vi "仁科测控通讯.vi"() -> ()   [LabVIEW 2016, in "环境动力监测库.lvlib" / "空调库.lvlib"]
uses:
  <vilib>/Plasmionique/MB Master/MB_Master/MB_Master.lvclass
  <vilib>/Plasmionique/MB Master/MB Master.lvlib
panel:
  out "运行状态":T1
  out "告警状态":T2
  out "传感器状态输出":T3
  out "温湿度解析":cluster{"湿度":dbl, "温度":dbl}
  out "系统参数":u16[](array[numeric])
  out "告警状态":u16[](array[numeric])
  out "传感器状态":u16[](array[numeric])
  out "温湿度解析":u16[](array[numeric])
  in  "读取数据":bool
  in  "释放串口":bool
  in  "打开串口":bool
  out "通讯状态":bool
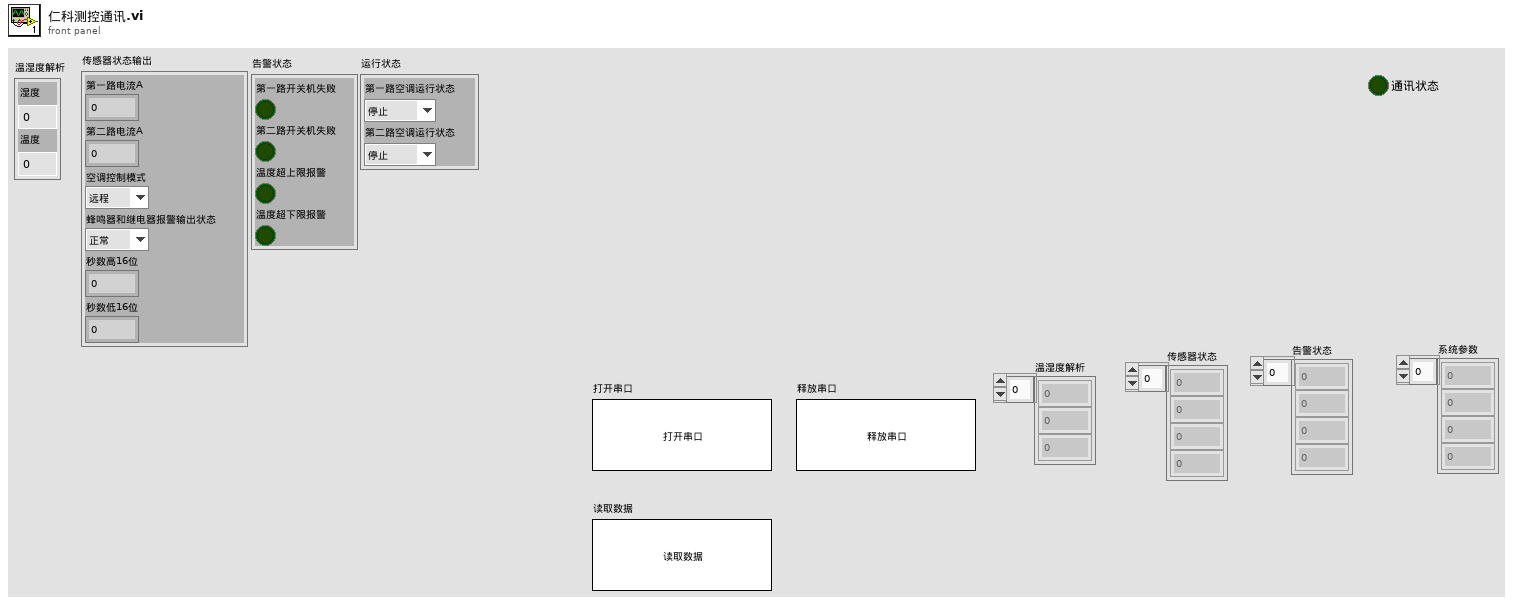
[diagram p1: front panel]
types:
  T1 = cluster{"第一路空调运行状态":enum16{"停止", "制冷", "制热", "未知"}, "第二路空调运行状态":enum16{"停止", "制冷", "制热", "未知"}}
  T2 = cluster{"第一路开关机失败":bool, "第二路开关机失败":bool, "温度超上限报警":bool, "温度超下限报警":bool}
  T3 = cluster{"第一路电流A":u16, "第二路电流A":u16, "空调控制模式":enum16{"远程", "自动"}, "蜂鸣器和继电器报警输出状态":enum16{"正常", "报警"}, "秒数高16位":u16, "秒数低16位":u16}
  T4 = cluster{"型号选择":enum16{"黑盾", "英维克", "仁科测控RS-KTC-N01"}, "MB session in":refnum<class "MB_Master.lvclass">, "英维克空调寄存器":u16[], "通讯状态":bool, "PORT":string, "IP":string, "Slave ID ":u8, "Serial Config":cluster{"baud rate (bps)":u32, "stop bits":u16, "parity":u16, "flow control":u16, "timeout":u32, "retries":i32}, "VISA Resource":refnum<visa-resource-name>, "MB通信方式选择":enum16{"串口", "TCP"}}
  T5 = enum16{"open", "read", "write single", "write", "close"}
  T6 = cluster{"温湿度解析":cluster{"湿度":dbl, "温度":dbl}, "传感器状态输出":cluster{"第一路电流A":u16, "第二路电流A":u16, "空调控制模式":enum16{"远程", "自动"}, "蜂鸣器和继电器报警输出状态":enum16{"正常", "报警"}, "秒数高16位":u16, "秒数低16位":u16}, "告警状态":cluster{"第一路开关机失败":bool, "第二路开关机失败":bool, "温度超上限报警":bool, "温度超下限报警":bool}, "运行状态":cluster{"第一路空调运行状态":enum16{"停止", "制冷", "制热", "未知"}, "第二路空调运行状态":enum16{"停止", "制冷", "制热", "未知"}}}
  T7 = cluster{"第一路电流":u16, "第二路电流":u16, "空调控制模式":enum16{"远程", "自动"}, "蜂鸣器和继电器报警输出状态":enum16{"正常", "报警"}, "秒数高16位":u16, "秒数低16位":u16}
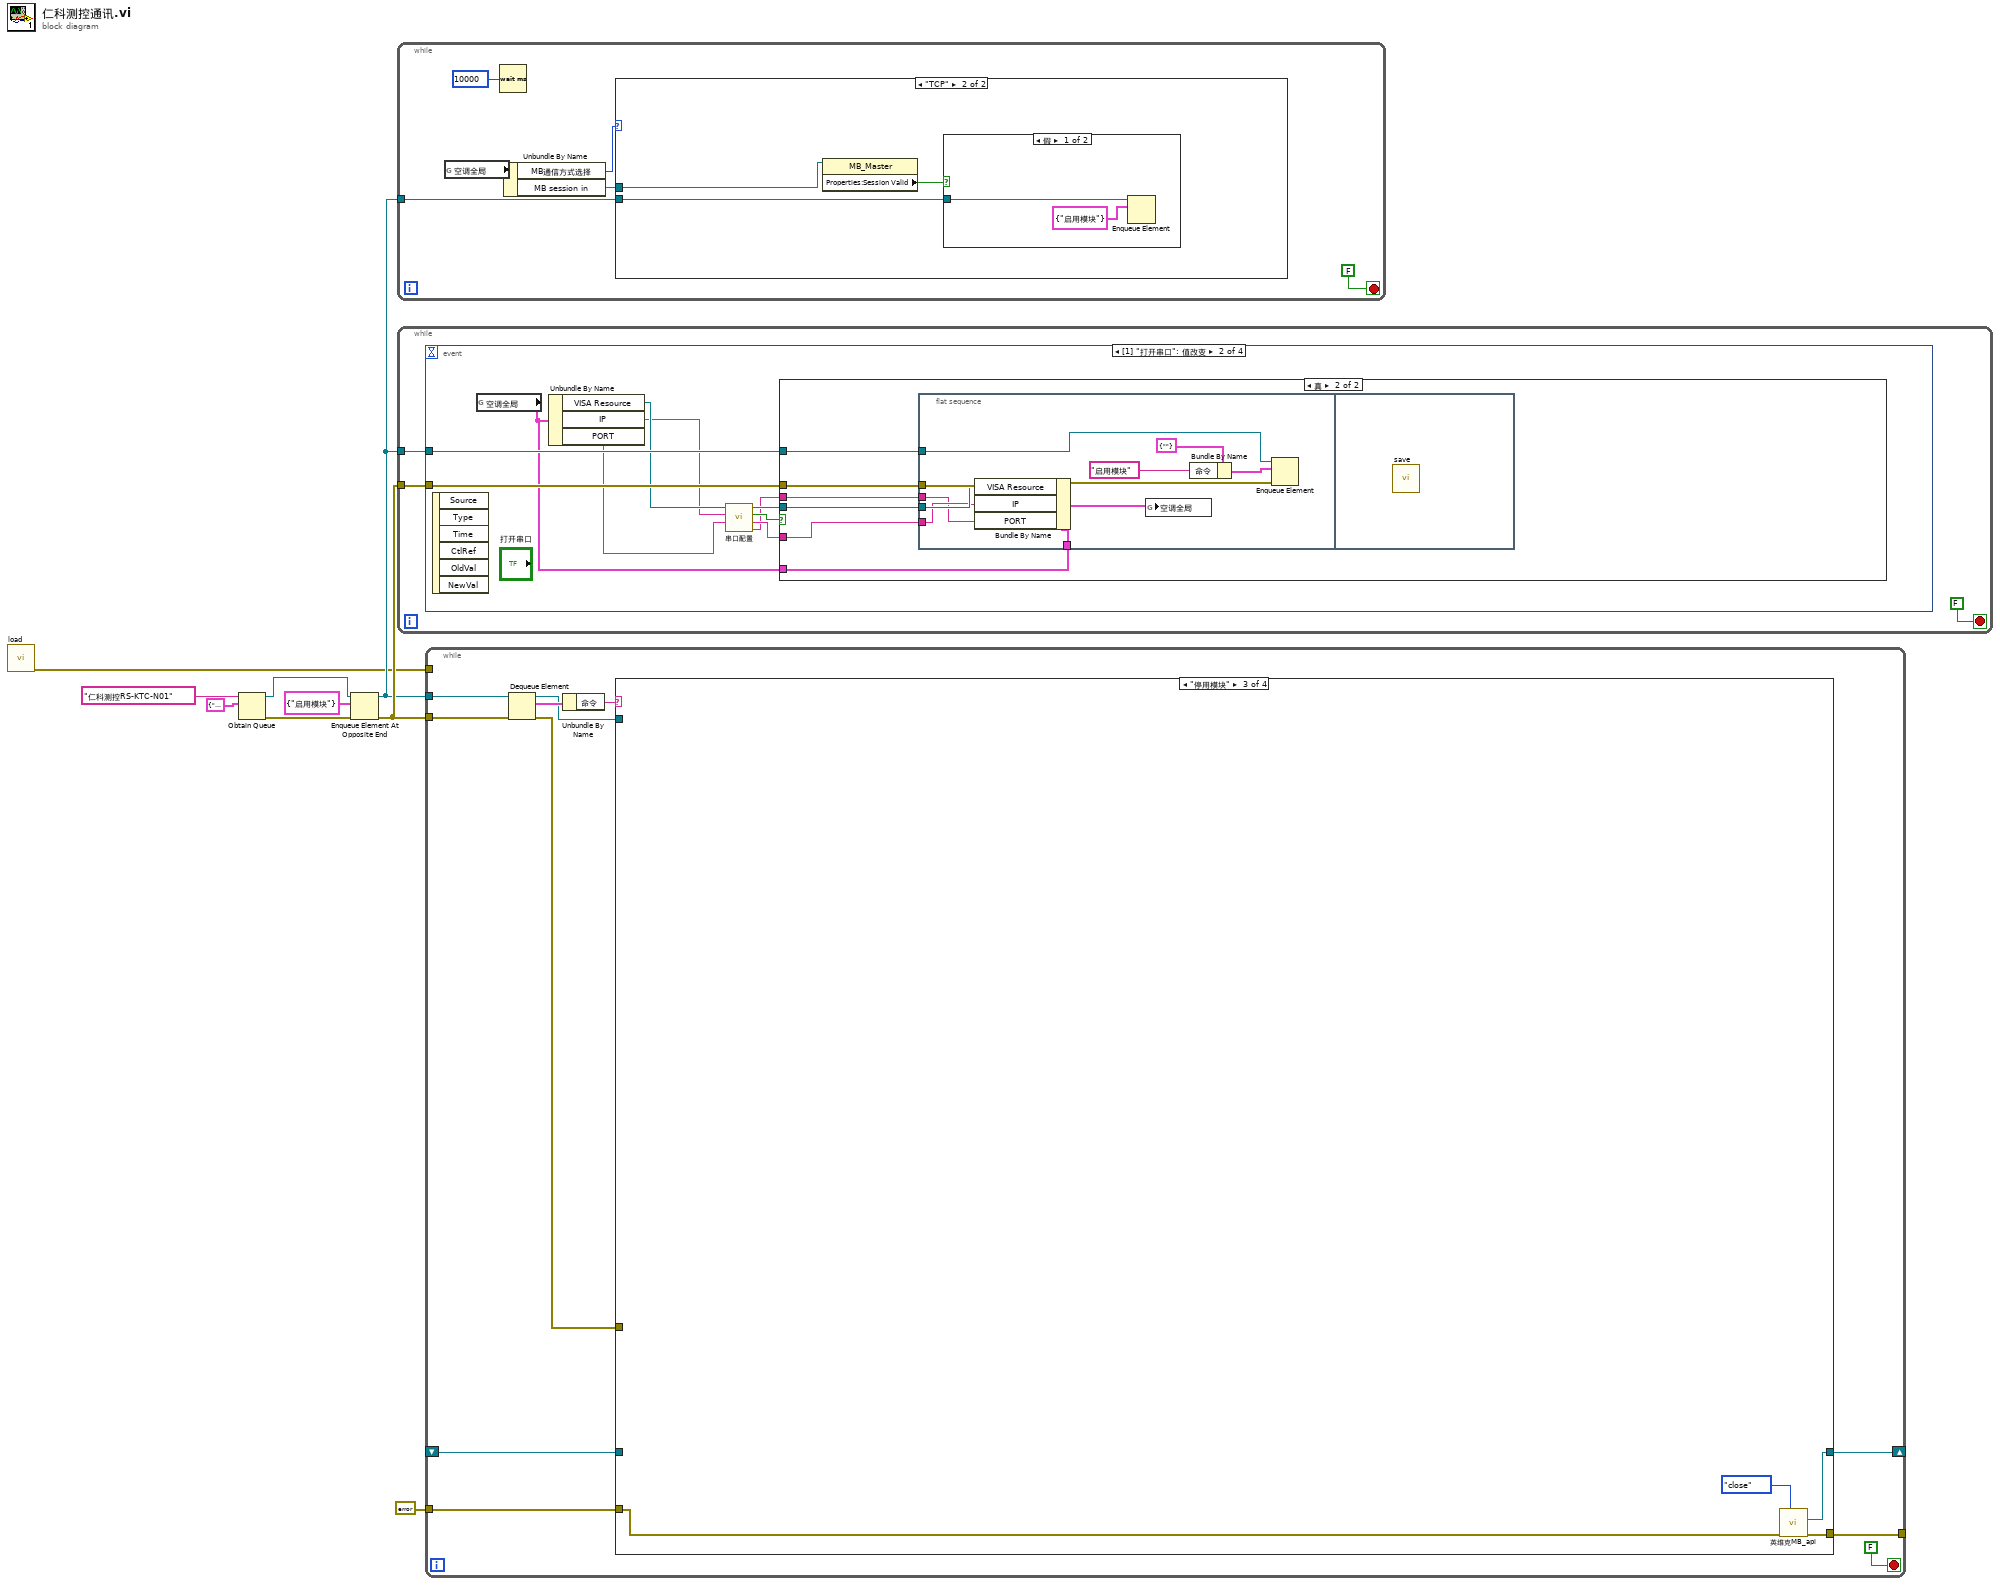
[diagram p0: block diagram]
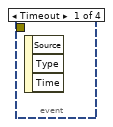
[diagram p4: hidden frame]
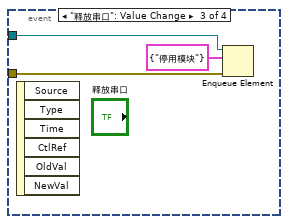
[diagram p6: hidden frame]
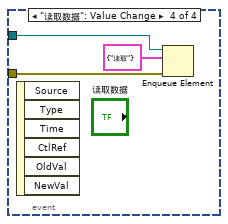
[diagram p7: hidden frame]
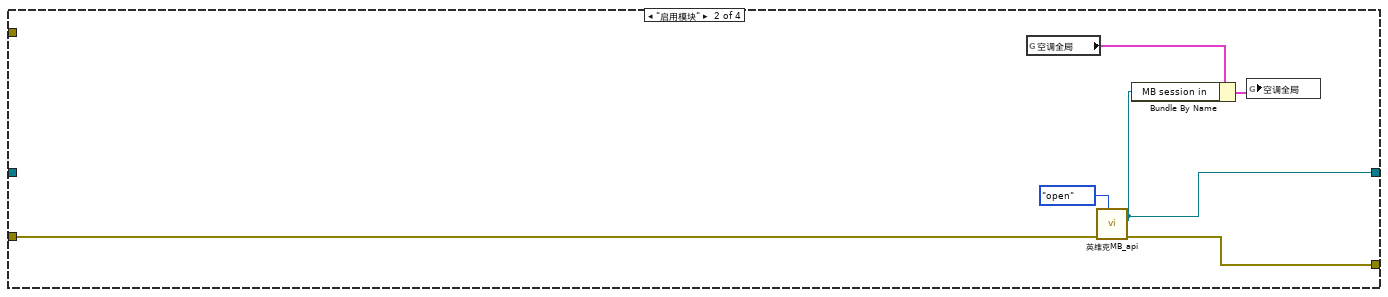
[diagram p9: hidden frame]
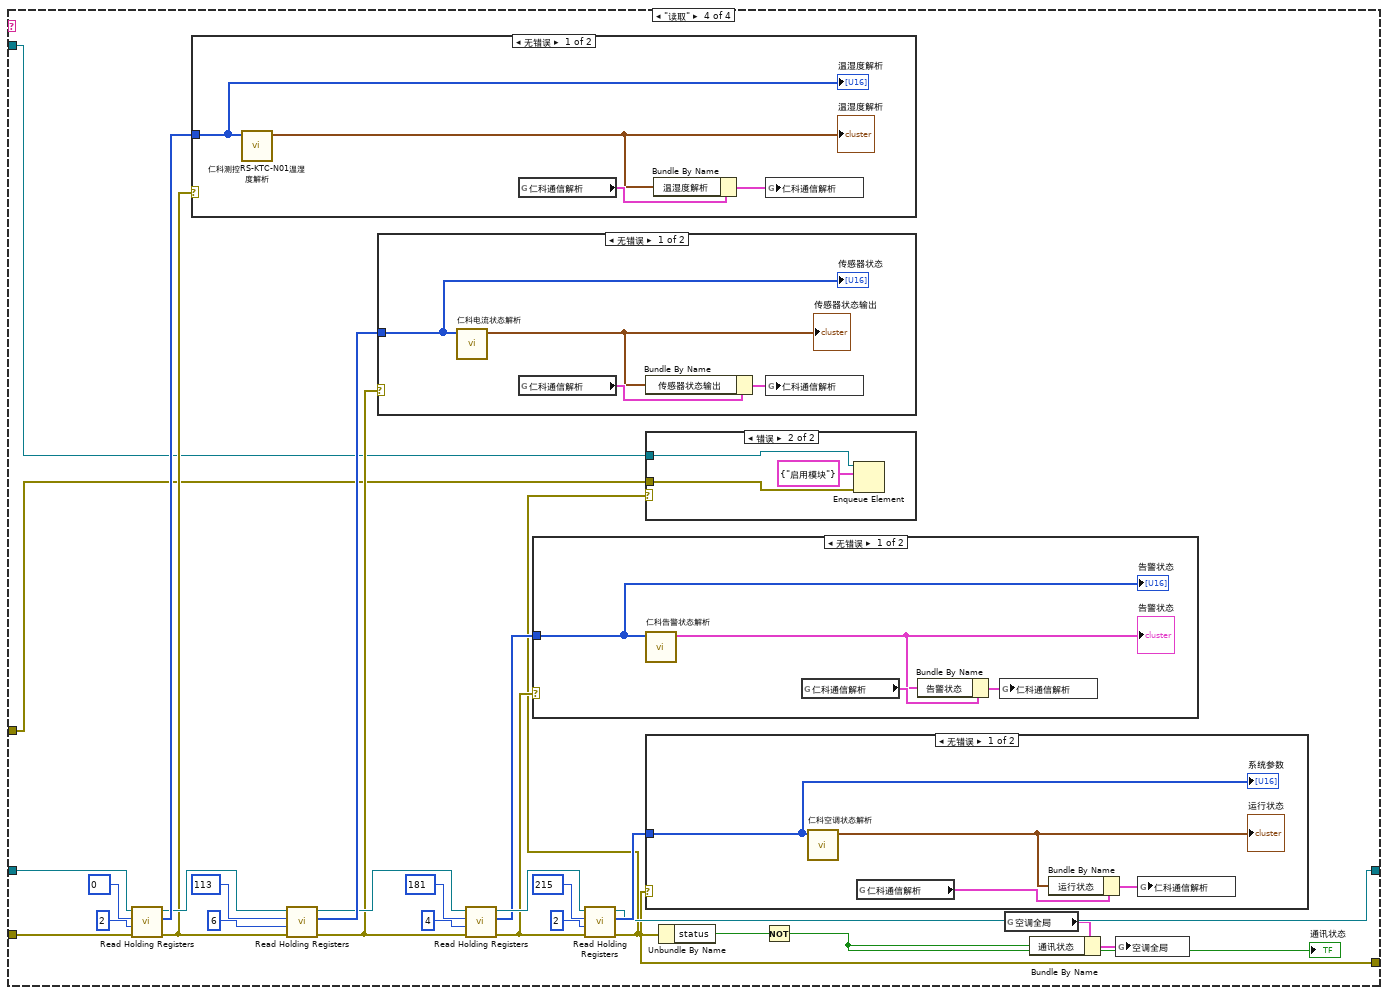
[diagram p10: hidden frame]
diagram:
  n1 = call "load.vi"() -> ("error out"=w1:errorcluster)  [unwired: 11 in]
  n2 = Obtain Queue(name (unnamed)="仁科测控RS-KTC-N01" ("名称（未命名）"), element data type=cluster{"命令":string} {"命令"="启用模块"} ("元素")) -> (queue out=w6:refnum<queue>, error out=w5:errorcluster)  [unwired: 3 in, 1 out]
  n3 = Enqueue Element At Opposite End(queue=w6, element=cluster{"命令":string} {"命令"="启用模块"} ("元素"), error in (no error)=w5) -> (queue out=w2:refnum<queue>, error out=w3:errorcluster)  [unwired: 1 in, 1 out]
  n4 = while {
    tunnel: w2 -> [w15]
    stop <- FALSE stop-if-true
    n5 = global read "断电保存全局变量.vi" "空调全局"() -> (w12:T4)
    n6 = Wait (ms)(milliseconds to wait=u32 10000 ("等待时间（毫秒）")) -> ()  [unwired: 1 out]
    n7 = Unbundle By Name(w12) -> ("MB通信方式选择"=w11:enum16{"串口", "TCP"}, "MB session in"=w10:refnum<class "MB_Master.lvclass">)
    n8 = case shown="\"TCP\"" w11 {
      tunnel: w15 -> [_ w17]
      tunnel: w10 -> [_ w16]
      frame "串口", Default {
      }
      frame "TCP" {
        n9 = property class="MB_Master"(reference=w16) -> ("Properties:Session Valid"=w18:bool)  [unwired: 1 in, 2 out]
        n10 = case shown="假" w18 {
          tunnel: w17 -> [w20 _]
          frame False {
            n11 = Enqueue Element(queue=w20, element=cluster{"命令":string} {"命令"="启用模块"} ("元素")) -> ()  [unwired: 2 in, 3 out]
          }
          frame True {
          }
        }
      }
    }
  }
  n12 = while {
    tunnel: w2 -> [w22]
    tunnel: w3 -> [w21]
    stop <- FALSE stop-if-true
    n13 = event shown="[1] \"打开串口\": 值改变" {
      selector: _ -> [_ _ _ _]
      dyn-events: _ -> [_ _ _ _]
      timeout: _ -> [_ _ _ _]
      tunnel: w22 -> [_ w33 w52 w54]
      tunnel: w21 -> [_ w32 w51 w53]
      event Timeout {
        n14 = event-data() -> ()  [unwired: 1 in, 3 out]
      }
      event "打开串口": Value Change {
        n15 = event-data() -> ()  [unwired: 1 in, 6 out]
        n16 = global read "断电保存全局变量.vi" "空调全局"() -> (w24:T4)
        n17 = Unbundle By Name(w24) -> ("VISA Resource"=w27:refnum<visa-resource-name>, "IP"=w26:string, "PORT"=w25:string)
        n18 = call "串口配置.vi"("PORT"=w25, "IP"=w26, "请选择串口:"=w27) -> ("PORT 2"=w28:string, "IP 2"=w29:string, "确认 2"=w30:bool, "VISA资源名称 2"=w31:refnum<visa-resource-name>)  [unwired: 5 in]
        n19 = case shown="真" w30 {
          tunnel: w31 -> [_ w37]
          tunnel: w33 -> [_ w39]
          tunnel: w32 -> [_ w38]
          tunnel: w29 -> [_ w36]
          tunnel: w28 -> [_ w35]
          tunnel: w24 -> [_ w34]
          frame False {
          }
          frame True {
            n20 = flat-sequence {
              tunnel: w39 -> [w46]
              tunnel: w38 -> [w45]
              tunnel: w37 -> [w42]
              tunnel: w36 -> [w41]
              tunnel: w35 -> [w40]
              tunnel: w34 -> [w44]
              frame #0 {
                n21 = Bundle By Name(cluster=w44, "VISA Resource"=w42, "IP"=w41, "PORT"=w40) -> (w43:T4)
                n22 = global write "断电保存全局变量.vi" "空调全局"(w43) -> ()
                n23 = Bundle By Name(cluster=cluster{"命令":string} {"命令"=""} ("元素"), "命令"="启用模块" ("名称（未命名）")) -> (w47:cluster{"命令":string})
                n24 = Enqueue Element(queue=w46, element=w47, error in (no error)=w45) -> ()  [unwired: 1 in, 3 out]
              }
              frame #1 {
                n25 = call "save.vi"() -> ()  [unwired: 11 in, 1 out]
              }
            }
          }
        }
      }
      event "释放串口": Value Change {
        n26 = event-data() -> ()  [unwired: 1 in, 6 out]
        n27 = Enqueue Element(queue=w52, element=cluster{"命令":string} {"命令"="停用模块"} ("元素"), error in (no error)=w51) -> ()  [unwired: 1 in, 3 out]
      }
      event "读取数据": Value Change {
        n28 = event-data() -> ()  [unwired: 1 in, 6 out]
        n29 = Enqueue Element(queue=w54, element=cluster{"命令":string} {"命令"="读取"} ("元素"), error in (no error)=w53) -> ()  [unwired: 1 in, 3 out]
      }
    }
  }
  n30 = while {
    tunnel: w2 -> [w58]
    tunnel: w3 -> [w65]
    tunnel: [w59] -> _
    shift-right: [w62] -> _
    shift-left: _ -> [w61]
    tunnel: errorcluster {"status"=FALSE, "code"=0, "source"=""} ("error out") -> [w60]
    tunnel: w1 -> [_]
    stop <- FALSE stop-if-true
    n31 = Dequeue Element(queue=w58, error in (no error)=w65) -> (queue out=w57:refnum<queue>, element=w64:cluster{"命令":string}, error out=w56:errorcluster)  [unwired: 1 in, 1 out]
    n32 = Unbundle By Name(w64) -> ("命令"=w63:string)
    n33 = case shown="\"停用模块\"" w63 {
      tunnel: [w68 w70 w76 w83] -> w62
      tunnel: [w67 w74 w77 w82] -> w59
      tunnel: w61 -> [w68 _ _ w106]
      tunnel: w60 -> [w67 w73 w78 w105]
      tunnel: w57 -> [_ _ _ w85]
      tunnel: w56 -> [_ _ _ w84]
      frame Default {
      }
      frame "启用模块" {
        n34 = global read "断电保存全局变量.vi" "空调全局"() -> (w71:T4)
        n35 = call "英维克MB_api.vi"("STEP"=T5."open", "Error in"=w73) -> ("error out"=w74:errorcluster, "MB session out"=w70:refnum<class "MB_Master.lvclass">)  [unwired: 7 in, 1 out]
        n36 = Bundle By Name(cluster=w71, "MB session in"=w70) -> (w69:T4)
        n37 = global write "断电保存全局变量.vi" "空调全局"(w69) -> ()
      }
      frame "停用模块" {
        n38 = call "英维克MB_api.vi"("STEP"=T5."close", "Error in"=w78) -> ("error out"=w77:errorcluster, "MB session out"=w76:refnum<class "MB_Master.lvclass">)  [unwired: 7 in, 1 out]
      }
      frame "读取" {
        n39 = call <vilib>:"Read Holding Registers.vi"("error in (no error)"=w105, "quantity"=u16 2 ("number of holding registers"), "starting address"=u16 0, "MB session in"=w106) -> ("error out"=w102:errorcluster, "Registers"=w104:u16[], "MB session out"=w103:refnum<class "MB_Master.lvclass">)  [unwired: 5 in]
        n40 = case shown="无错误" w102 {
          tunnel: w104 -> [w125 _]
          frame No Error {
            n41 = call "仁科测控RS-KTC-N01温湿度解析.vi"("运行状态输入"=w125) -> ("温湿度解析"=w122:cluster{"湿度":dbl, "温度":dbl})  [unwired: 10 in]
            "温湿度解析" <- w122
            n42 = global read "内部交互全局变量.vi" "仁科通信解析"() -> (w124:T6)
            n43 = Bundle By Name(cluster=w124, "温湿度解析"=w122) -> (w123:T6)
            n44 = global write "内部交互全局变量.vi" "仁科通信解析"(w123) -> ()
            "温湿度解析" <- w125
          }
          frame Error {
          }
        }
        n45 = call <vilib>:"Read Holding Registers.vi"("error in (no error)"=w102, "quantity"=u16 6 ("number of holding registers"), "starting address"=u16 113, "MB session in"=w103) -> ("error out"=w94:errorcluster, "Registers"=w101:u16[], "MB session out"=w95:refnum<class "MB_Master.lvclass">)  [unwired: 5 in]
        n46 = case shown="无错误" w94 {
          tunnel: w101 -> [w121 _]
          frame No Error {
            n47 = call "仁科电流状态解析.vi"("传感器状态输入"=w121) -> ("传感器状态输出"=w118:T7)  [unwired: 10 in]
            "传感器状态输出" <- w118
            n48 = global read "内部交互全局变量.vi" "仁科通信解析"() -> (w120:T6)
            n49 = Bundle By Name(cluster=w120, "传感器状态输出"=w118) -> (w119:T6)
            n50 = global write "内部交互全局变量.vi" "仁科通信解析"(w119) -> ()
            "传感器状态" <- w121
          }
          frame Error {
          }
        }
        n51 = call <vilib>:"Read Holding Registers.vi"("error in (no error)"=w94, "quantity"=u16 4 ("number of holding registers"), "starting address"=u16 181, "MB session in"=w95) -> ("error out"=w88:errorcluster, "Registers"=w87:u16[], "MB session out"=w89:refnum<class "MB_Master.lvclass">)  [unwired: 5 in]
        n52 = case shown="无错误" w88 {
          tunnel: w87 -> [w117 _]
          frame No Error {
            n53 = call "仁科告警状态解析.vi"("告警状态输入"=w117) -> ("告警状态"=w114:T2)  [unwired: 10 in]
            "告警状态" <- w114
            n54 = global read "内部交互全局变量.vi" "仁科通信解析"() -> (w116:T6)
            n55 = Bundle By Name(cluster=w116, "告警状态"=w114) -> (w115:T6)
            n56 = global write "内部交互全局变量.vi" "仁科通信解析"(w115) -> ()
            "告警状态" <- w117
          }
          frame Error {
          }
        }
        n57 = call <vilib>:"Read Holding Registers.vi"("error in (no error)"=w88, "quantity"=u16 2 ("number of holding registers"), "starting address"=u16 215, "MB session in"=w89) -> ("error out"=w82:errorcluster, "Registers"=w86:u16[], "MB session out"=w83:refnum<class "MB_Master.lvclass">)  [unwired: 5 in]
        n58 = case shown="错误" w82 {
          tunnel: w85 -> [_ w109]
          tunnel: w84 -> [_ w107]
          frame No Error {
          }
          frame Error {
            n59 = Enqueue Element(queue=w109, element=cluster{"命令":string} {"命令"="启用模块"} ("元素"), error in (no error)=w107) -> ()  [unwired: 1 in, 3 out]
          }
        }
        n60 = case shown="无错误" w82 {
          tunnel: w86 -> [w113 _]
          frame No Error {
            n61 = call "仁科空调状态解析.vi"("系统参数输入"=w113) -> ("运行状态"=w110:T1)  [unwired: 10 in]
            "运行状态" <- w110
            n62 = global read "内部交互全局变量.vi" "仁科通信解析"() -> (w112:T6)
            n63 = Bundle By Name(cluster=w112, "运行状态"=w110) -> (w111:T6)
            n64 = global write "内部交互全局变量.vi" "仁科通信解析"(w111) -> ()
            "系统参数" <- w113
          }
          frame Error {
          }
        }
        n65 = Unbundle By Name(w82) -> ("status"=w96:bool)
        n66 = Not(x=w96) -> (.not. x?=w79:bool)
        "通讯状态" <- w79
        n67 = global read "断电保存全局变量.vi" "空调全局"() -> (w80:T4)
        n68 = Bundle By Name(cluster=w80, "通讯状态"=w79) -> (w81:T4)
        n69 = global write "断电保存全局变量.vi" "空调全局"(w81) -> ()
      }
    }
  }
